vi "Enable.vi"(8 "error in (no error)":errorcluster, 11 "DC Brick in":refnum<class "DC Brick.lvclass">) -> (0 "error out":errorcluster, 3 "DC Brick out":refnum<class "DC Brick.lvclass">)   [LabVIEW 2011, in "Tinkerforge.lvlib" / "DC Brick.lvclass"]
doc: "This VI enables the motor. The motor can be configured (velocity, acceleration, etc) before it is enabled."
uses:
  DC Brick.lvclass
  Device/Device.lvclass
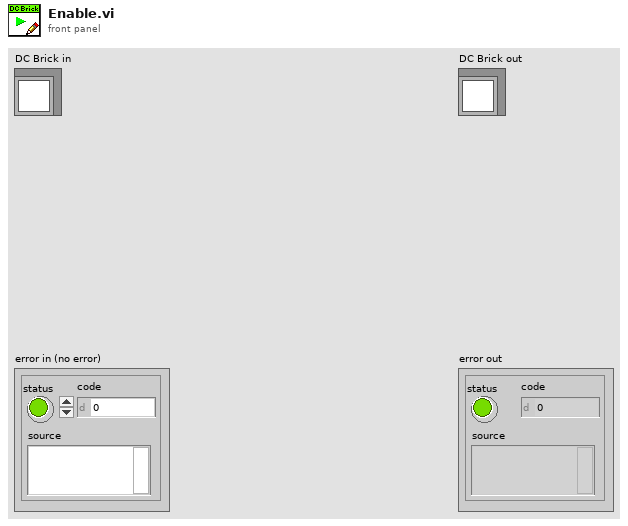
[diagram p1: front panel]
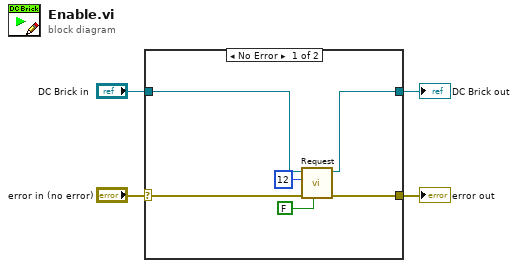
[diagram p0: block diagram]
diagram:
  n1 = case shown="No Error" "error in (no error)" {
    selector: "error in (no error)" -> [w5 w12]
    tunnel: [w6 w12] -> w3
    tunnel: [w9 w11] -> w1
    tunnel: "DC Brick in" -> [w10 w11]
    frame No Error {
      n2 = call "Request.vi"("Response"=FALSE, "error in (no error)"=w5, "Function ID"=u8 12, "Device in"=w10) -> ("error out"=w6:errorcluster, "Device out"=w9:refnum<class "DC Brick.lvclass">)  [unwired: 3 in, 3 out]
    }
    frame Error {
    }
  }
  "error out" <- w3
  "DC Brick out" <- w1
